vi "Forebrain.vi"() -> ()   [LabVIEW 2012]
uses:
  <vilib>/Utility/inputDevices.llb/closeKeyboard.vi
  <vilib>/Utility/inputDevices.llb/keyboardAcquire.vi
panel:
  out "error out":errorcluster
  out "Simulation UDP":bool
  out "Heading":i32
  in  "MANUAL \nOVERRIDE":bool
  out "Starboard Speed":i32(knob) scale=1000.0..2000.0
  out "Port Speed":i32(knob) scale=1000.0..2000.0
  in  "Rudders":i32(slide)=1500 scale=500.0..2500.0
  in  "Step Size":i32=5
  out "Speed                    Balance":i32(knob) scale=-1000.0..1000.0
  in  "Pan Camera":i32(slide)=1500 scale=500.0..2500.0
  in  "FULL STOP":bool
  out "UDP Timeout":bool
  out "UDP Working":bool
  in  "ESTOP":bool
  in  "PC Status":i32=1
  out "Port Rudder":i32
  out "Starboard Rudder":i32
  out "Port Motor":i32
  out "Starboard Motor":i32
  out "Data from XBEE":dbl
  out "XBEE Working":bool
  out "return count":u32
  out "Sent from XBEE":string
  out "bytes written":u32
  in  "Send to XBEE":string
  in  "VISA resource name":refnum<visa-resource-name>="COM6"
  in  "error in":errorcluster
  out "Base Station data rec'd":string
  out "Robot Stats":i32[](array[numeric])
  out "Buoy locations":cluster{"regular expression":string, i32, i32}[](array[cluster])
  # "ORGANIZE FRONT PANEL"
  # "Tug X"
  # "Tug Y"
  # "Tug H"
  # "MANUAL OVERRIDE CONTROLS"
  # "Controls:\nUse W/S to independently\ncontrol port speed.\nUse I/K to independently\ncontrol starboard speed.\nUse arrow keys to jointly\ncontrol motor speeds.\n\nUSE ESCAPE TO KILL MOTORS."
  # "Affects weight of single key input."
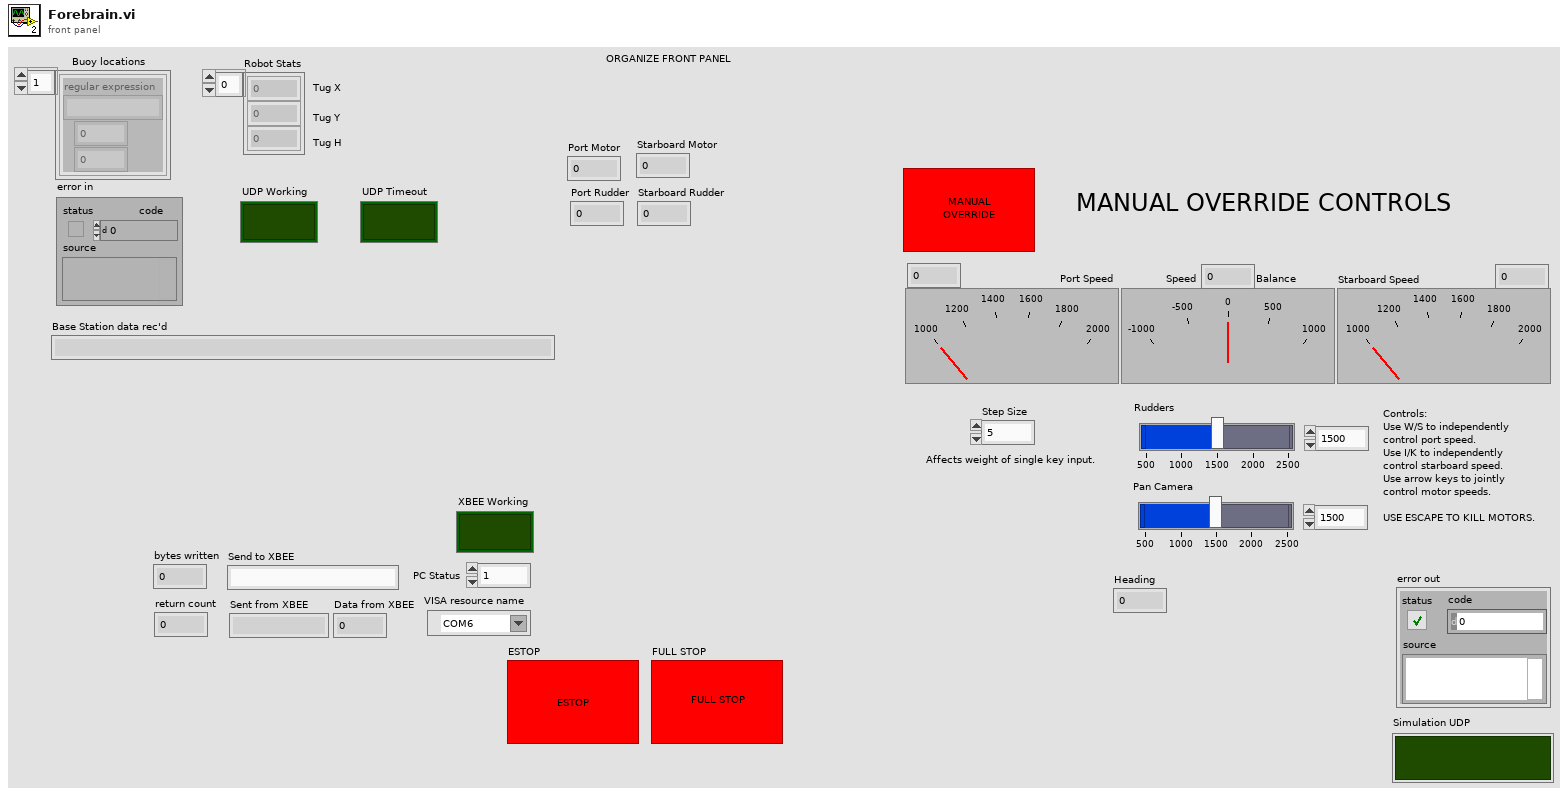
[diagram p1: front panel]
types:
  T1 = enum16{"0", "1", "2", "3", "4", "5", "6", "7", "8", "9", "A", "B", "C", "D", "E", "F", "G", "H", "I", "J", "K", "L", "M", "N", "O", "P", "Q", "R", "S", "T", "U", "V", "W", "X", "Y", "Z", "F1", "F2", "F3", "F4", "F5", "F6", "F7", "F8", "F9", "F10", "F11", "F12", "F13", "F14", "F15", "ADD", "BACK", "BACKSLASH", "CAPITAL", "COMMA", "DECIMAL", "DELETE", "DIVIDE", "DOWN", "END", "EQUALS", "ESCAPE", "GRAVE (`)", "HOME", "INSERT", "LBRACKET", "LCONTROL", "LEFT", "L ALT", "LSHIFT", "LWIN", "MINUS", "MULTIPLY", "NEXT", "NUMLOCK", "NUMPAD_0", "NUMPAD_1", "NUMPAD_2", "NUMPAD_3", "NUMPAD_4", "NUMPAD_5", "NUMPAD_6", "NUMPAD_7", "NUMPAD_8", "NUMPAD_9", "PAUSE", "PERIOD", "PRIOR (PG UP)", "RBRACKET", "RCONTROL", "RETURN", "RIGHT", "R ALT", "RSHIFT", "RWIN", "SCROLL", "SEMICOLON", "SLASH", "SPACE", "SUBTRACT", "TAB", "UP", "ENTER (num pad)", "' (quote)"}[]
  T2 = enum16{"0", "1", "2", "3", "4", "5", "6", "7", "8", "9", "A", "B", "C", "D", "E", "F", "G", "H", "I", "J", "K", "L", "M", "N", "O", "P", "Q", "R", "S", "T", "U", "V", "W", "X", "Y", "Z", "F1", "F2", "F3", "F4", "F5", "F6", "F7", "F8", "F9", "F10", "F11", "F12", "F13", "F14", "F15", "ADD", "BACK", "BACKSLASH", "CAPITAL", "COMMA", "DECIMAL", "DELETE", "DIVIDE", "DOWN", "END", "EQUALS", "ESCAPE", "GRAVE (`)", "HOME", "INSERT", "LBRACKET", "LCONTROL", "LEFT", "L ALT", "LSHIFT", "LWIN", "MINUS", "MULTIPLY", "NEXT", "NUMLOCK", "NUMPAD_0", "NUMPAD_1", "NUMPAD_2", "NUMPAD_3", "NUMPAD_4", "NUMPAD_5", "NUMPAD_6", "NUMPAD_7", "NUMPAD_8", "NUMPAD_9", "PAUSE", "PERIOD", "PRIOR (PG UP)", "RBRACKET", "RCONTROL", "RETURN", "RIGHT", "R ALT", "RSHIFT", "RWIN", "SCROLL", "SEMICOLON", "SLASH", "SPACE", "SUBTRACT", "TAB", "UP", "ENTER (num pad)", "' (quote)"}
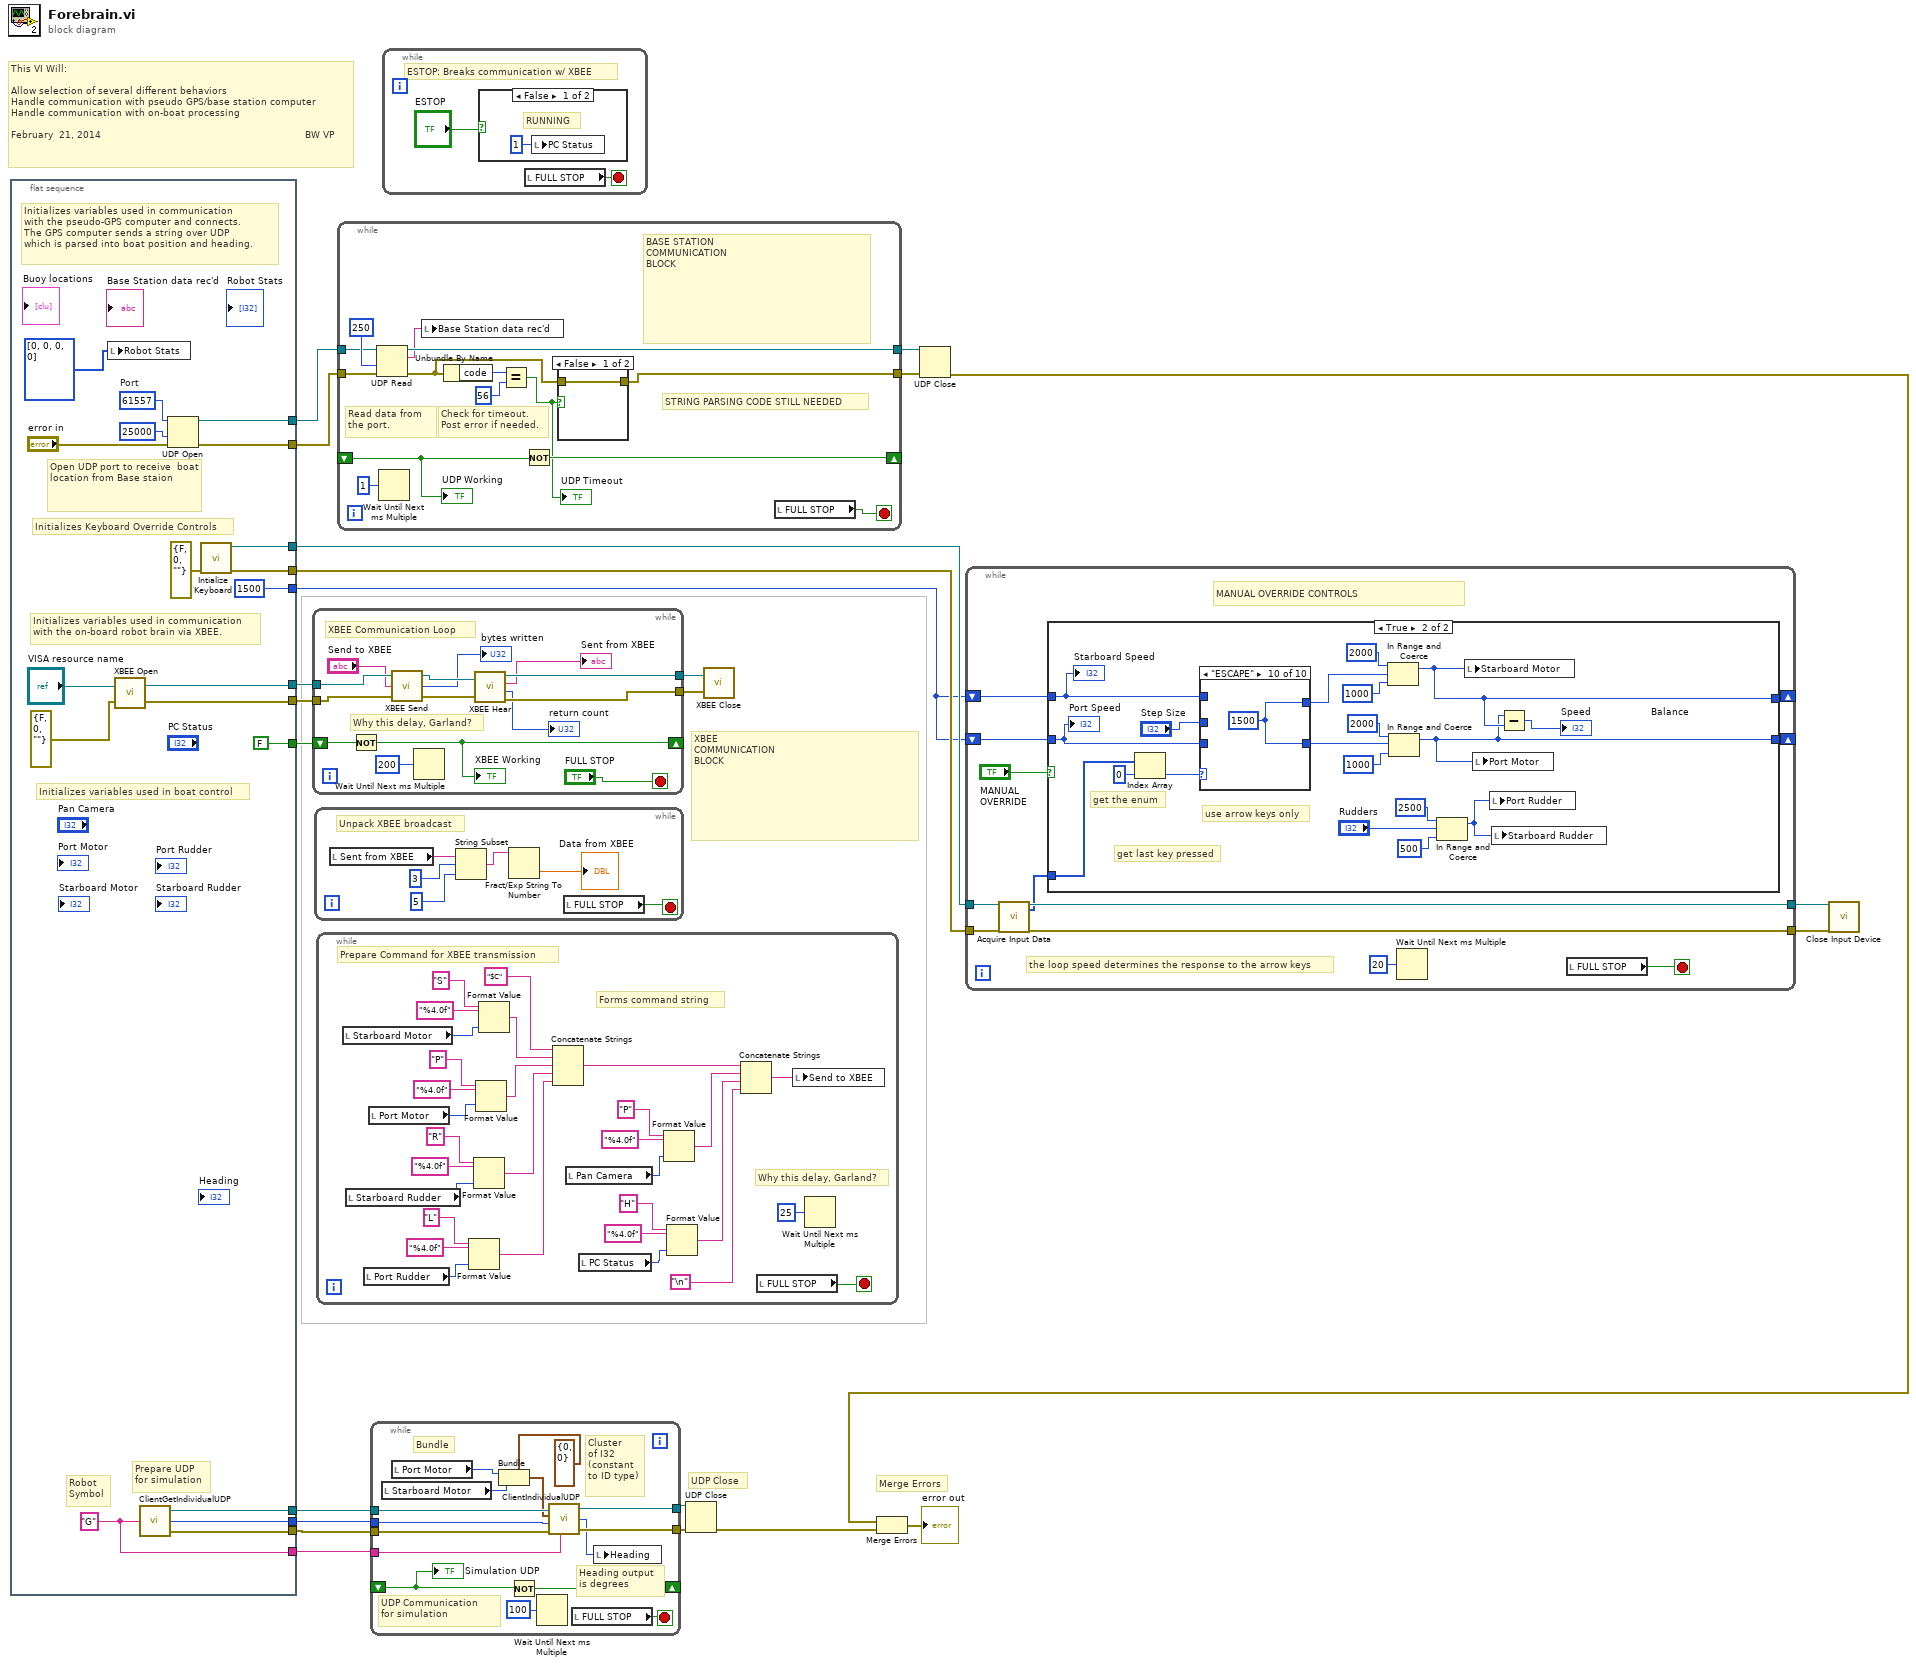
[diagram p0: block diagram]
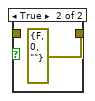
[diagram p2: hidden frame]
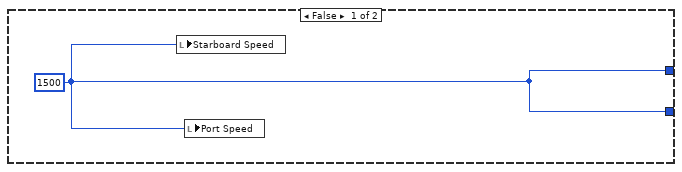
[diagram p3: hidden frame]
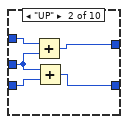
[diagram p5: hidden frame]
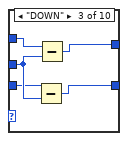
[diagram p6: hidden frame]
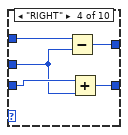
[diagram p7: hidden frame]
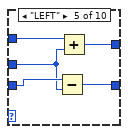
[diagram p8: hidden frame]
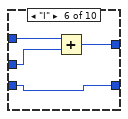
[diagram p9: hidden frame]
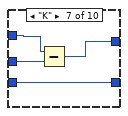
[diagram p10: hidden frame]
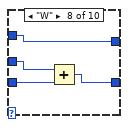
[diagram p11: hidden frame]
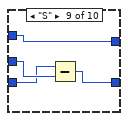
[diagram p12: hidden frame]
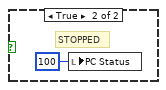
[diagram p13: hidden frame]
diagram:
  # "Merge Errors"
  # "UDP Close"
  # "XBEE \nCOMMUNICATION\nBLOCK"
  # "This VI Will:\n\nAllow selection of several different behaviors\nHandle communication with pseudo GPS/base station computer\nHandle communication with on-boat processing\n\nFebruary  21, 2014                                                                    BW VP"
  n1 = flat-sequence {
    tunnel: [w38] -> w12
    tunnel: [w37] -> w11
    tunnel: [w34] -> w23
    tunnel: [w33] -> w22
    tunnel: [FALSE] -> w19
    tunnel: [w30] -> w17
    tunnel: [w29] -> w16
    tunnel: [1500] -> w15
    tunnel: [w27] -> w6
    tunnel: [w26] -> w5
    tunnel: [w25] -> w4
    tunnel: [w24] -> w3
    frame #0 {
      w24 = "G"
      w41 = u16 61557  # Port
      # "Prepare UDP\nfor simulation"
      # "Robot \nSymbol"
      # "Initializes Keyboard Override Controls"
      # "Initializes variables used in boat control"
      # "Initializes variables used in communication\nwith the on-board robot brain via XBEE."
      # "Initializes variables used in communication\nwith the pseudo-GPS computer and connects.\nThe GPS computer sends a string over UDP\nwhich is parsed into boat position and heading."
      # "Open UDP port to receive  boat location from Base staion"
      n2 = local write "Robot Stats"(i32[] [0, 0, 0, 0]) -> ()
      n3 = call "XBEE Open.vi"("error in"=errorcluster {"status"=FALSE, "code"=0, "source"=""}, "VISA resource name"="VISA resource name") -> ("error out"=w33:errorcluster, "VISA resource name out"=w34:refnum<visa-resource-name>)
      n4 = call "ClientGetIndividualUDP.vi"("Robot Symbol"=w24) -> ("UDP Connection ID"=w27:refnum<k16>, "Remote Port #"=w26:i32, "error out"=w25:errorcluster)
      n5 = UDP Open(8:"error in", 9:25000 ("timeout ms (25000)"), 11:w41) -> (port=w38:refnum<k16>, 0:w37:errorcluster)  [unwired: 2 in, 1 out]
      n6 = call <vilib>:"Intialize Keyboard.vi"("error in (no error)"=errorcluster {"status"=FALSE, "code"=0, "source"=""}) -> ("error out"=w29:errorcluster, "device ID"=w30:refnum<k1>)  [unwired: 9 in]
    }
  }
  n7 = while {
    tunnel: w23 -> [w56]
    tunnel: w22 -> [w55]
    tunnel: [w50] -> w21
    tunnel: [w49] -> w20
    shift-right: [w44] -> _
    shift-left: w19 -> [w46]
    stop <- "FULL STOP" stop-if-true
    # "Why this delay, Garland?"
    # "XBEE Communication Loop"
    n8 = Not(x=w46) -> (.not. x?=w44:bool)
    "XBEE Working" <- w44
    n9 = call "XBEE Send.vi"("error in (no error)"=w55, "String"="Send to XBEE", "VISA resource name"=w56) -> ("error out"=w52:errorcluster, "return count"=→"bytes written":u32, "VISA resource name out"=w53:refnum<visa-resource-name>)
    n10 = Wait Until Next ms Multiple(millisecond multiple=200) -> ()  [unwired: 1 out]
    n11 = call "XBEE Hear.vi"("VISA resource name"=w53, "error in (no error)"=w52) -> ("VISA resource name out"=w50:refnum<visa-resource-name>, "String Received"=→"Sent from XBEE":string, "return count"=→"return count":u32, "error out"=w49:errorcluster)
  }
  n12 = while {
    stop <- w62 stop-if-true
    # "Unpack XBEE broadcast"
    n13 = local read "Sent from XBEE"() -> (w61:string)
    n14 = String Subset(string=w61, offset (0)=3, length (rest)=5 ("length (rest)")) -> (substring=w58:string)
    n15 = Fract/Exp String To Number(string=w58) -> (number=→"Data from XBEE":dbl)  [unwired: 3 in, 1 out]
    n16 = local read "FULL STOP"() -> (w62:bool)
  }
  n17 = while {
    stop <- w92 stop-if-true
    # "Why this delay, Garland?"
    # "Prepare Command for XBEE transmission"
    # "Forms command string"
    n18 = local read "Starboard Motor"() -> (w89:i32)
    n19 = local read "Starboard Rudder"() -> (w80:i32)
    n20 = local read "Port Rudder"() -> (w77:i32)
    n21 = local read "Port Motor"() -> (w86:i32)
    n22 = Format Value(string ("")="L", format string="%4.0f", value (0)=w77) -> (output string=w75:string)
    n23 = Format Value(string ("")="R", format string="%4.0f", value (0)=w80) -> (output string=w76:string)
    n24 = Format Value(string ("")="P", format string="%4.0f", value (0)=w86) -> (output string=w83:string)
    n25 = Format Value(string ("")="S", format string="%4.0f", value (0)=w89) -> (output string=w84:string)
    n26 = Concatenate Strings("$C", w84, w83, w76, w75) -> (w67:string)
    n27 = local read "Pan Camera"() -> (w71:i32)
    n28 = local read "PC Status"() -> (w68:i32)
    n29 = Format Value(string ("")="P", format string="%4.0f", value (0)=w71) -> (output string=w66:string)
    n30 = Format Value(string ("")="H", format string="%4.0f", value (0)=w68) -> (output string=w65:string)
    n31 = Concatenate Strings(w67, w66, w65, "\n") -> (w72:string)
    n32 = local read "FULL STOP"() -> (w92:bool)
    n33 = local write "Send to XBEE"(w72) -> ()
    n34 = Wait Until Next ms Multiple(millisecond multiple=u32 25) -> ()  [unwired: 1 out]
  }
  n35 = while {
    shift-right: [w104] -> _
    shift-left: _ -> [w94]
    tunnel: [w103] -> w14
    tunnel: [w99] -> w13
    tunnel: w12 -> [w97]
    tunnel: w11 -> [w96]
    stop <- w95 stop-if-true
    # "BASE STATION \nCOMMUNICATION\nBLOCK"
    # "Check for timeout.\nPost error if needed."
    # "Read data from\nthe port."
    # "STRING PARSING CODE STILL NEEDED"
    n36 = UDP Read(connection ID=w97, timeout ms (25000)=250, 8:w96) -> (data out=w98:string, error out=w100:errorcluster, 3:w103:refnum<k16>)  [unwired: 1 in, 2 out]
    n37 = Wait Until Next ms Multiple(millisecond multiple=u32 1) -> ()  [unwired: 1 out]
    n38 = local write "Base Station data rec'd"(w98) -> ()
    n39 = Unbundle By Name(w100) -> ("code"=w102:i32)
    n40 = Equal?(x=w102, y=56) -> (x = y?=w93:bool)
    "UDP Timeout" <- w93
    n41 = Not(x=w94) -> (.not. x?=w104:bool)
    n42 = case shown="False" w93 {
      tunnel: w100 -> [w107 _]
      tunnel: [w107 errorcluster {"status"=FALSE, "code"=0, "source"=""} ("error out")] -> w99
      frame False {
      }
      frame True {
      }
    }
    n43 = local read "FULL STOP"() -> (w95:bool)
    "UDP Working" <- w94
  }
  n44 = while {
    tunnel: w3 -> [w123]
    tunnel: w4 -> [w122]
    tunnel: w6 -> [w121]
    tunnel: w5 -> [w120]
    tunnel: [w115] -> w9
    tunnel: [w114] -> w10
    shift-right: [w111] -> _
    shift-left: _ -> [w110]
    stop <- w112 stop-if-true
    # "UDP Communication \nfor simulation"
    # "Heading output\nis degrees"
    # "Cluster\nof I32\n(constant\nto ID type)"
    # "Bundle"
    n45 = local read "Starboard Motor"() -> (w118:i32)
    n46 = local read "Port Motor"() -> (w119:i32)
    n47 = Bundle(cluster=cluster{i32, i32} {0, 0}, w119, w118) -> (w117:cluster{i32, i32})
    n48 = Not(x=w110) -> (.not. x?=w111:bool)
    n49 = Wait Until Next ms Multiple(millisecond multiple=u32 100) -> ()  [unwired: 1 out]
    n50 = call "ClientIndividualUDP.vi"("UDP Connection ID"=w121, "Rover Inputs"=w117, "Remote Port #"=w120, "error in (no error)"=w122, "Robot Symbol"=w123) -> ("connection ID out"=w115:refnum<k16>, "Robot Heading"=w113:i32, "error out"=w114:errorcluster)
    n51 = local read "FULL STOP"() -> (w112:bool)
    n52 = local write "Heading"(w113) -> ()
    "Simulation UDP" <- w110
  }
  n53 = while {
    stop <- w125 stop-if-true
    # "ESTOP: Breaks communication w/ XBEE"
    n54 = case shown="False" "ESTOP" {
      frame False {
        # "RUNNING"
        n55 = local write "PC Status"(1 ("PC Status")) -> ()
      }
      frame True {
        # "STOPPED"
        n56 = local write "PC Status"(100) -> ()
      }
    }
    n57 = local read "FULL STOP"() -> (w125:bool)
  }
  n58 = UDP Close(connection ID=w9, 8:w10) -> (error out=w7:errorcluster)  [unwired: 1 out]
  n59 = call "XBEE Close.vi"("error in (no error)"=w20, "VISA resource name"=w21) -> ()
  n60 = UDP Close(connection ID=w14, 8:w13) -> (error out=w1:errorcluster)  [unwired: 1 out]
  n61 = Merge Errors(w1, w7) -> (→"error out":errorcluster)
  n62 = while {
    tunnel: [w139] -> w2
    tunnel: [w138] -> w18
    shift-right: [w132] -> _
    shift-left: w15 -> [w135]
    shift-right: [w131] -> _
    shift-left: w15 -> [w134]
    tunnel: w17 -> [w130]
    tunnel: w16 -> [w129]
    stop <- w133 stop-if-true
    # "MANUAL OVERRIDE CONTROLS"
    # "the loop speed determines the response to the arrow keys"
    n63 = call-poly <vilib>:"Acquire Input Data.vi"("device ID"=w130, "error in (no error)"=w129) -> ("device ID"=w138:refnum<k1>, "keys pressed"=w137:T1, "error out"=w139:errorcluster)  [unwired: 15 in]
    n64 = case shown="True" "MANUAL \nOVERRIDE" {
      tunnel: w137 -> [_ w159]
      tunnel: w135 -> [_ w156]
      tunnel: w134 -> [_ w155]
      tunnel: [w140 w143] -> w132
      tunnel: [w140 w142] -> w131
      frame False {
        w140 = 1500
        n65 = local write "Starboard Speed"(w140) -> ()
        n66 = local write "Port Speed"(w140) -> ()
      }
      frame True {
        # "use arrow keys only"
        # "get the enum"
        # "get last key pressed"
        n67 = Index Array(array=w159, index=0) -> (element=w157:T2)
        n68 = case shown="\"ESCAPE\"" w157 {
          tunnel: w156 -> [w161 w166 w171 w173 w178 w185 w187 w190 w194 _]
          tunnel: [w161 w165 w170 w174 w179 w184 w186 w190 w194 w198] -> w154
          tunnel: w155 -> [w160 w163 w168 w176 w180 w182 w189 w192 w196 _]
          tunnel: [w160 w162 w167 w175 w181 w182 w189 w191 w195 w198] -> w145
          tunnel: "Step Size" -> [_ w164 w169 w172 w177 w183 w188 w193 w197 _]
          frame "0", Default {
          }
          frame "UP" {
            n69 = Add(x=w166, y=w164) -> (x+y=w165:i32)
            n70 = Add(x=w164, y=w163) -> (x+y=w162:i32)
          }
          frame "DOWN" {
            n71 = Subtract(x=w168, y=w169) -> (x-y=w167:i32)
            n72 = Subtract(x=w171, y=w169) -> (x-y=w170:i32)
          }
          frame "RIGHT" {
            n73 = Subtract(x=w173, y=w172) -> (x-y=w174:i32)
            n74 = Add(x=w176, y=w172) -> (x+y=w175:i32)
          }
          frame "LEFT" {
            n75 = Subtract(x=w180, y=w177) -> (x-y=w181:i32)
            n76 = Add(x=w178, y=w177) -> (x+y=w179:i32)
          }
          frame "I" {
            n77 = Add(x=w185, y=w183) -> (x+y=w184:i32)
          }
          frame "K" {
            n78 = Subtract(x=w187, y=w188) -> (x-y=w186:i32)
          }
          frame "W" {
            n79 = Add(x=w193, y=w192) -> (x+y=w191:i32)
          }
          frame "S" {
            n80 = Subtract(x=w196, y=w197) -> (x-y=w195:i32)
          }
          frame "ESCAPE" {
            w198 = 1500
          }
        }
        n81 = In Range and Coerce(upper limit=2000, x=w154, lower limit=1000) -> (coerced(x)=w143:i32)  [unwired: 1 out]
        n82 = In Range and Coerce(upper limit=2000, x=w145, lower limit=1000) -> (coerced(x)=w142:i32)  [unwired: 1 out]
        n83 = In Range and Coerce(upper limit=2500, x="Rudders", lower limit=500) -> (coerced(x)=w141:i32)  [unwired: 1 out]
        n84 = local write "Starboard Motor"(w143) -> ()
        n85 = local write "Port Motor"(w142) -> ()
        n86 = local write "Port Rudder"(w141) -> ()
        n87 = local write "Starboard Rudder"(w141) -> ()
        n88 = Subtract(x=w142, y=w143) -> (x-y=→"Speed                    Balance":i32)
        "Starboard Speed" <- w156
        "Port Speed" <- w155
      }
    }
    n89 = Wait Until Next ms Multiple(millisecond multiple=u32 20) -> ()  [unwired: 1 out]
    n90 = local read "FULL STOP"() -> (w133:bool)
  }
  n91 = call-poly <vilib>:"Close Input Device.vi"("error in (no error)"=w2, "device ID"=w18) -> ()  [unwired: 8 in, 1 out]
